vi "Read Time.vi"(8 "error in (no error)":errorcluster, 10 "Shutter-NP":T1, 11 "Container in":refnum<class "Container.lvclass">) -> (0 "error out":errorcluster, 2 "Shutter-NP out":T1, 3 "Container out":refnum<class "Container.lvclass">)   [LabVIEW 2016, in "Container.lvclass"]
uses:
  Container.lvclass
  Controls/Shutters.ctl
  Controls/Shutter Data.ctl
  Controls/Shutter States.ctl
  Container.lvclass/Container.ctl
  Sci/SciShutt.lvclass
  LFCSim/LFCSimShutt.lvclass
  ExtFlat/ExtFlatShutt.lvclass
  SimFlat/SimFlatShutt.lvclass
  Solar/SolarShutt.lvclass
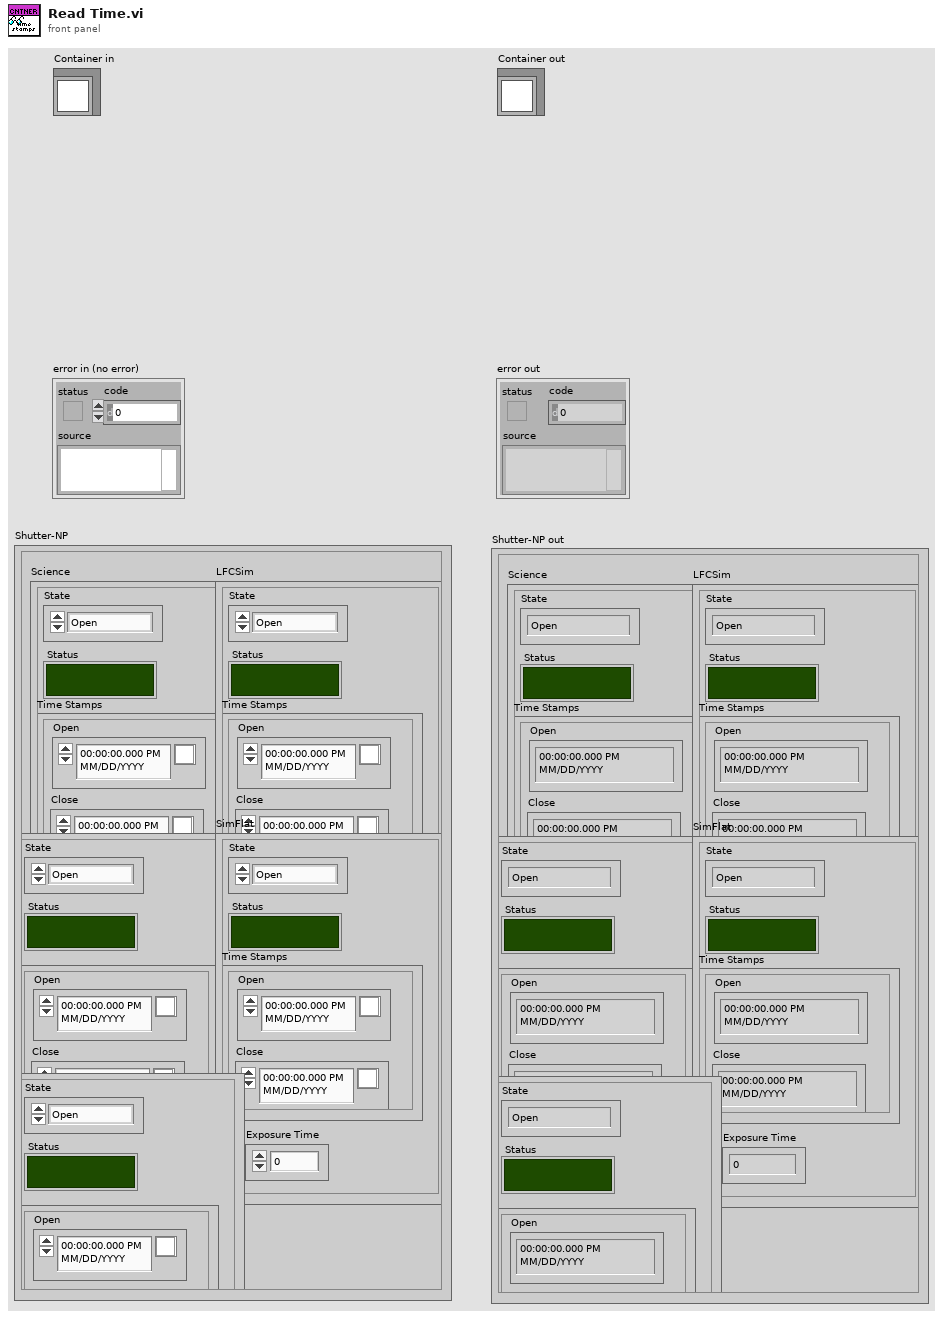
[diagram p1: front panel]
types:
  T1 = typedef "Shutters.ctl" = cluster{"Science":T2, "LFCSim":T2, "ExtendFlat":T2, "SimFlat":T2, "Solar":T2}
  T2 = typedef "Shutter Data.ctl" = cluster{"Status":bool, "State":T3, "Time Stamps":cluster{"Open":timestamp, "Close":timestamp}, "Exposure Time":dbl}
  T3 = typedef "Shutter States.ctl" = enum16{"Open", "Close", "Wait", "Off", "Arm", "Idle"}
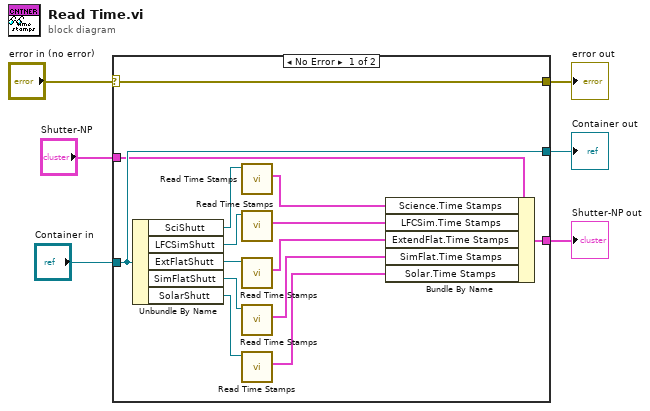
[diagram p0: block diagram]
diagram:
  n1 = case shown="No Error" "error in (no error)" {
    selector: "error in (no error)" -> [w20 w22]
    tunnel: [w20 w22] -> w5
    tunnel: [w19 w23] -> w3
    tunnel: "Container in" -> [w19 w23]
    tunnel: "Shutter-NP" -> [w17 w21]
    tunnel: [w18 w21] -> w1
    frame No Error {
      n2 = Unbundle By Name(w19) -> ("SciShutt"=w16:refnum<class "SciShutt.lvclass">, "LFCSimShutt"=w14:refnum<class "LFCSimShutt.lvclass">, "ExtFlatShutt"=w13:refnum<class "ExtFlatShutt.lvclass">, "SimFlatShutt"=w12:refnum<class "SimFlatShutt.lvclass">, "SolarShutt"=w11:refnum<class "SolarShutt.lvclass">)
      n3 = call-dynamic "Read Time Stamps.vi"("Shutter in"=w16) -> ("Time Stamps"=w15:cluster{"Open":timestamp, "Close":timestamp})  [unwired: 8 in, 2 out]
      n4 = call-dynamic "Read Time Stamps.vi"("Shutter in"=w14) -> ("Time Stamps"=w10:cluster{"Open":timestamp, "Close":timestamp})  [unwired: 8 in, 2 out]
      n5 = call-dynamic "Read Time Stamps.vi"("Shutter in"=w13) -> ("Time Stamps"=w9:cluster{"Open":timestamp, "Close":timestamp})  [unwired: 8 in, 2 out]
      n6 = call-dynamic "Read Time Stamps.vi"("Shutter in"=w12) -> ("Time Stamps"=w8:cluster{"Open":timestamp, "Close":timestamp})  [unwired: 8 in, 2 out]
      n7 = call-dynamic "Read Time Stamps.vi"("Shutter in"=w11) -> ("Time Stamps"=w7:cluster{"Open":timestamp, "Close":timestamp})  [unwired: 8 in, 2 out]
      n8 = Bundle By Name(cluster=w17, "Science.Time Stamps"=w15, "LFCSim.Time Stamps"=w10, "ExtendFlat.Time Stamps"=w9, "SimFlat.Time Stamps"=w8, "Solar.Time Stamps"=w7) -> (w18:T1)
    }
    frame Error {
    }
  }
  "error out" <- w5
  "Container out" <- w3
  "Shutter-NP out" <- w1
